vi "Diode_Sweep.vi"() -> ()   [LabVIEW 2019]
panel:
  out "Napiecie na diodzie [V]":dbl
  out "Nr pomiaru":i32
  out "read buffer 4":string
  out "XY Graph":cluster{"X":dbl[], "Y":dbl[]}[](graph)
  out "Boolean 2":bool
  out "Boolean":bool
  out "Prad [A]":dbl
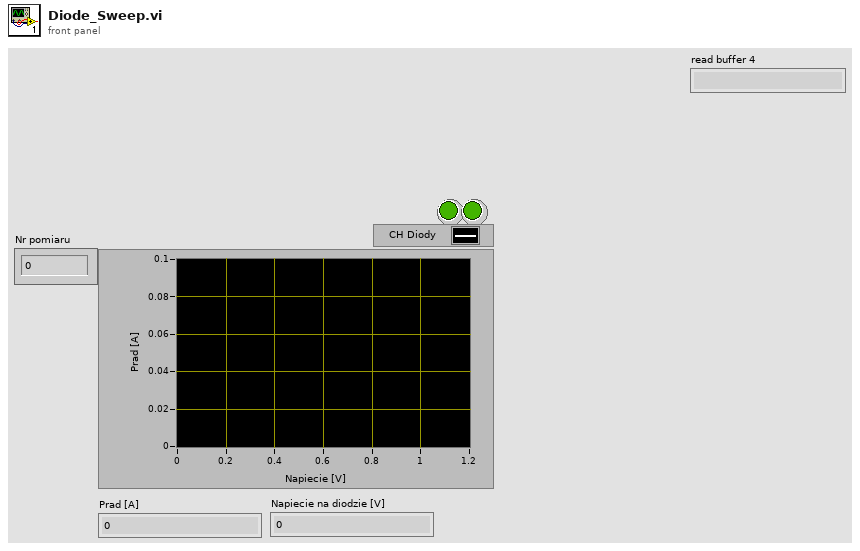
[diagram p1: front panel]
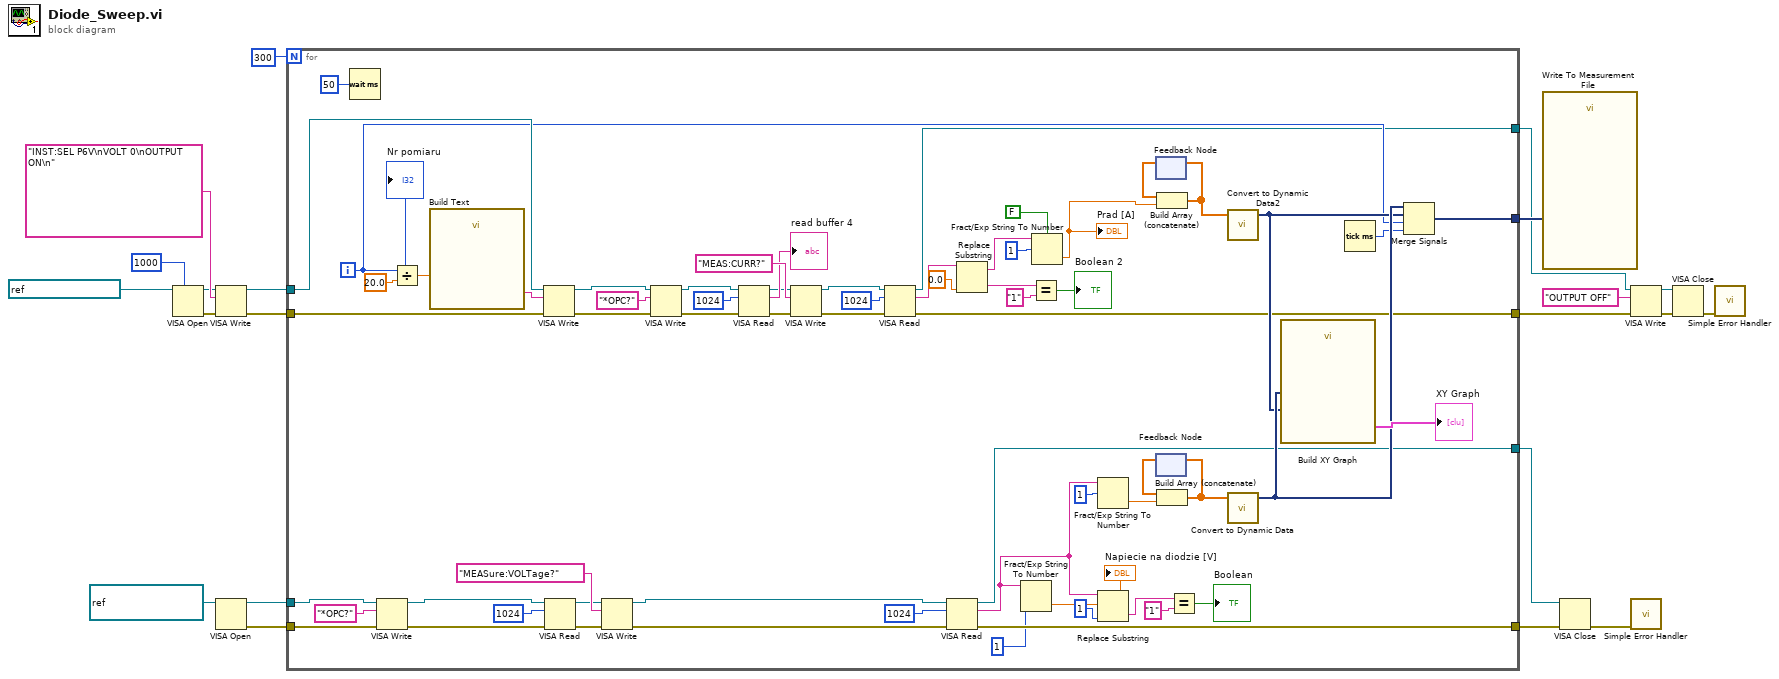
[diagram p0: block diagram]
diagram:
  n1 = VISA Open(timeout (0)=u32 1000 ("VISA Open timeout (0)"), VISA resource name=refnum<visa-resource-name> "GPIB0::9::INSTR") -> (VISA resource name=w14:refnum<visa-resource-name>, error out=w16:errorcluster)  [unwired: 3 in]
  n2 = VISA Write(VISA resource name=w14, write buffer="INST:SEL P6V\nVOLT 0\nOUTPUT ON\n", error in (no error)=w16) -> (VISA resource name out=w12:refnum<visa-resource-name>, error out=w13:errorcluster)  [unwired: 1 out]
  n3 = VISA Open(VISA resource name=refnum<visa-resource-name> "GPIB0::10::INSTR") -> (VISA resource name=w21:refnum<visa-resource-name>, error out=w20:errorcluster)  [unwired: 4 in]
  n4 = for {
    N: 300 -> [_]
    tunnel: w21 -> [w34]
    tunnel: w20 -> [w33]
    tunnel: w13 -> [w59]
    tunnel: w12 -> [w58]
    tunnel: [w50] -> w11
    tunnel: [w38] -> w9
    tunnel: [w37] -> w7
    tunnel: [w28] -> w4
    tunnel: [w27] -> w3
    i -> [w52]
    n5 = Wait (ms)(milliseconds to wait=u32 50) -> ()  [unwired: 1 out]
    n6 = VISA Write(VISA resource name=w34, write buffer="*OPC?", error in (no error)=w33) -> (VISA resource name out=w36:refnum<visa-resource-name>, error out=w35:errorcluster)  [unwired: 1 out]
    n7 = Divide(x=w52, y=20.0) -> (x/y=w70:dbl)
    n8 = call "Build Text"("d"=w70) -> ("Result"=w62:string)  [unwired: 13 in, 1 out]
    n9 = VISA Write(VISA resource name=w58, write buffer=w62, error in (no error)=w59) -> (VISA resource name out=w43:refnum<visa-resource-name>, error out=w45:errorcluster)  [unwired: 1 out]
    n10 = VISA Read(VISA resource name=w36, byte count=u32 1024, error in (no error)=w35) -> (VISA resource name out=w30:refnum<visa-resource-name>, error out=w29:errorcluster)  [unwired: 2 out]
    n11 = VISA Write(VISA resource name=w30, write buffer="MEASure:VOLTage?", error in (no error)=w29) -> (VISA resource name out=w32:refnum<visa-resource-name>, error out=w31:errorcluster)  [unwired: 1 out]
    n12 = VISA Write(VISA resource name=w43, write buffer="*OPC?", error in (no error)=w45) -> (VISA resource name out=w42:refnum<visa-resource-name>, error out=w41:errorcluster)  [unwired: 1 out]
    n13 = VISA Read(VISA resource name=w42, byte count=u32 1024, error in (no error)=w41) -> (VISA resource name out=w39:refnum<visa-resource-name>, read buffer=→"read buffer 4":string, error out=w40:errorcluster)  [unwired: 1 out]
    n14 = VISA Write(VISA resource name=w39, write buffer="MEAS:CURR?", error in (no error)=w40) -> (VISA resource name out=w26:refnum<visa-resource-name>, error out=w56:errorcluster)  [unwired: 1 out]
    n15 = VISA Read(VISA resource name=w26, byte count=u32 1024, error in (no error)=w56) -> (VISA resource name out=w37:refnum<visa-resource-name>, read buffer=w60:string, error out=w38:errorcluster)  [unwired: 1 out]
    n16 = VISA Read(VISA resource name=w32, byte count=u32 1024, error in (no error)=w31) -> (VISA resource name out=w27:refnum<visa-resource-name>, read buffer=w24:string, error out=w28:errorcluster)  [unwired: 1 out]
    n17 = Replace Substring(2:0.0, 5:w60) -> (0:w82:string, 1:w83:string)  [unwired: 2 in]
    n18 = Fract/Exp String To Number(string=w24, offset=1) -> (number=→"Napiecie na diodzie [V]":dbl)  [unwired: 2 in, 1 out]
    n19 = Equal?(x=w82, y="1") -> (x = y?=→"Boolean 2":bool)
    n20 = Fract/Exp String To Number(use system decimal point (T)=FALSE, string=w83, offset=1) -> (number=w64:dbl)  [unwired: 1 in, 1 out]
    "Prad [A]" <- w64
    n21 = Fract/Exp String To Number(string=w24, offset=1) -> (number=w66:dbl)  [unwired: 2 in, 1 out]
    n22 = Replace Substring(2:1 ("length (len. of substring)"), 5:w24) -> (0:w84:string)  [unwired: 2 in, 1 out]
    n23 = feedback #1() -> (w65:dbl[])  [unwired: 1 in]
    n24 = feedback #2() -> (w67:dbl[])  [unwired: 1 in]
    n25 = Build Array (concatenate)(w65, w64) -> (w63:dbl[])
    n26 = feedback-in #1(w63) -> ()
    n27 = Build Array (concatenate)(w67, w66) -> (w68:dbl[])
    n28 = feedback-in #2(w68) -> ()
    n29 = Equal?(x=w84, y="1") -> (x = y?=→"Boolean":bool)
    n30 = call "Convert to Dynamic Data2"("Array"=w63) -> ("Dynamic Data Type"=w53:dynamicdata)  [unwired: 3 in]
    n31 = call "Convert to Dynamic Data"("Array"=w68) -> ("Dynamic Data Type"=w54:dynamicdata)  [unwired: 3 in]
    n32 = call "Build XY Graph"("Y Input"=w53, "X Input"=w54) -> ("XY Graph"=→"XY Graph":cluster{"X":dbl[], "Y":dbl[]}[])  [unwired: 8 in, 1 out]
    n33 = Tick Count (ms)() -> (millisecond timer value=w51:u32)
    n34 = Merge Signals(w54, w53, w52, w51) -> (w50:dynamicdata)
    "Nr pomiaru" <- w52
  }
  n35 = call "Write To Measurement File"("Signals"=w11) -> ()  [unwired: 16 in, 3 out]
  n36 = VISA Close(VISA resource name=w3, error in (no error)=w4) -> (error out=w2:errorcluster)
  n37 = VISA Write(VISA resource name=w7, write buffer="OUTPUT OFF", error in (no error)=w9) -> (VISA resource name out=w5:refnum<visa-resource-name>, error out=w6:errorcluster)  [unwired: 1 out]
  n38 = call <vilib>:"Simple Error Handler.vi"("error in (no error)"=w2) -> ()  [unwired: 4 in, 5 out]
  n39 = VISA Close(VISA resource name=w5, error in (no error)=w6) -> (error out=w10:errorcluster)
  n40 = call <vilib>:"Simple Error Handler.vi"("error in (no error)"=w10) -> ()  [unwired: 4 in, 5 out]
